vi "Build Hierarch Generator Recursive Call.vi"(0 "Node":refnum<data-value>, 1 "Working Set":refnum<data-value>, 11 "error in (no error)":errorcluster) -> (4 "Data Value Reference out":refnum<data-value>, 15 "error out":errorcluster)   [LabVIEW 2017, in "CL_G3_VIComponentBuilder.lvlib" / "Build Analyzer.lvclass"]
doc: "The recursive call that enables top down analysis."
uses:
  Build Analyzer.lvclass
  <userlib>/_Cirrus Logic/LabVIEW Container/Source/Container/Container.lvclass
  <userlib>/_Cirrus Logic/LabVIEW Container/Source/Container/Get Child.vi
  <userlib>/_Cirrus Logic/LabVIEW Container/Source/Container/Get All Attributes.vi
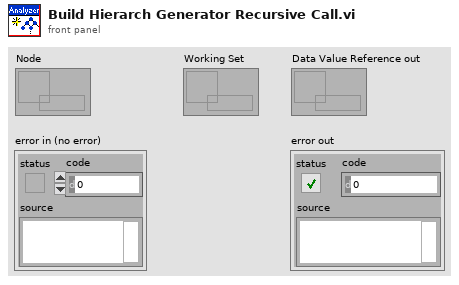
[diagram p1: front panel]
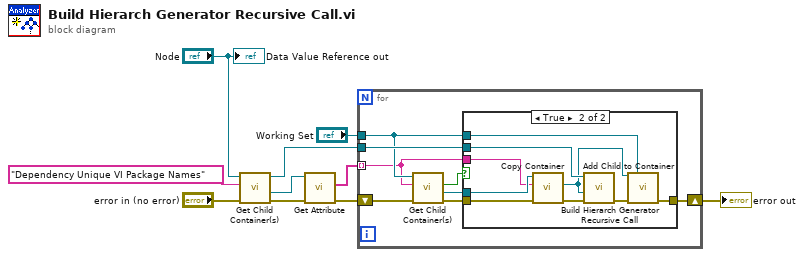
[diagram p0: block diagram]
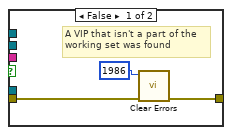
[diagram p2: hidden frame]
diagram:
  n1 = call-poly <userlib>:"Get Child Container(s).vi"("error in (no error)"="error in (no error)", "Container Name"="Dependency Unique VI Package Names", "Container"="Node") -> ("error out"=w4:errorcluster, "Child Container"=w8:refnum<data-value>, "dup Container"=w5:refnum<data-value>)  [unwired: 5 in, 1 out]
  n2 = call-poly <userlib>:"Get Attribute.vi"("error in (no error)"=w4, "Container"=w8) -> ("error out"=w3:errorcluster, "Attribute Names"=w10:string[])  [unwired: 6 in, 2 out]
  n3 = for {
    tunnel: w10 -> [w15] mode=indexing
    tunnel: "Working Set" -> [w17]
    tunnel: w5 -> [w18]
    shift-right: [w12] -> w1
    shift-left: w3 -> [w13]
    n4 = call-poly <userlib>:"Get Child Container(s).vi"("error in (no error)"=w13, "Container Name"=w15, "Container"=w17) -> ("error out"=w11:errorcluster, "Child Container"=w16:refnum<data-value>, "Container Found?"=w14:bool)  [unwired: 5 in, 1 out]
    n5 = case shown="True" w14 {
      tunnel: w18 -> [_ w29]
      tunnel: w17 -> [_ w28]
      tunnel: w16 -> [_ w27]
      tunnel: w15 -> [_ w25]
      tunnel: w11 -> [w20 w22]
      tunnel: [w19 w23] -> w12
      frame False {
        # "A VIP that isn't a part of the\nworking set was found"
        n6 = call <vilib>:"Clear Errors.vi"("error in (no error)"=w20, "specific error code to clear (0: all)"=1986) -> ("error out"=w19:errorcluster)  [unwired: 4 in, 1 out]
      }
      frame True {
        n7 = call <userlib>:"Copy Container.vi"("error in (no error)"=w22, "New Container Name"=w25, "Container"=w27) -> ("error out"=w24:errorcluster, "New Container"=w26:refnum<data-value>)  [unwired: 6 in, 1 out]
        n8 = call <userlib>:"Add Child to Container.vi"("error in (no error)"=w24, "Child Container"=w26, "Container"=w29) -> ("error out"=w30:errorcluster)  [unwired: 6 in, 2 out]
        n9 = call "Build Hierarch Generator Recursive Call.vi"("Node"=w26, "Working Set"=w28, "error in (no error)"=w30) -> ("error out"=w23:errorcluster)  [unwired: 11 in, 1 out]
      }
    }
  }
  "error out" <- w1
  "Data Value Reference out" <- "Node"
